vi "sequence_edited2.vi"() -> ()   [LabVIEW 2020]
uses:
  C:/Users/Public/Documents/Photometrics/PMQI-LabViewSamples/Examples/2018/Dependencies/PVCamNET.dll
  Dependencies/PVCamNET.dll
panel:
  in  "Trigger In Behaviour":string(combo)
  in  "Trigger Out Behaviour":string(combo)
  in  "Path":path
  out "SavingPath":string
  out "Boolean":bool
  in  "?":bool
  out "Capturing":bool
  in  "?":bool
  in  "FramesToCapture":u16
  in  "Exposure":u32
  in  "?":bool
  # "Description:\nThis code lets the user use sequence mode and save a TIFF image with \nthe user's preferred buffer size (framesToCapture) and exposure time. \n\nSteps to run:\n1. Update Path (Example: d:\\Temp\\ )\n2. Click \"Run\"\n3. Enter FramesToCapture and Exposure time\n4. Click \"START\"\n5. Click \"SAVE\"\n6. Click \"CLOSE\""
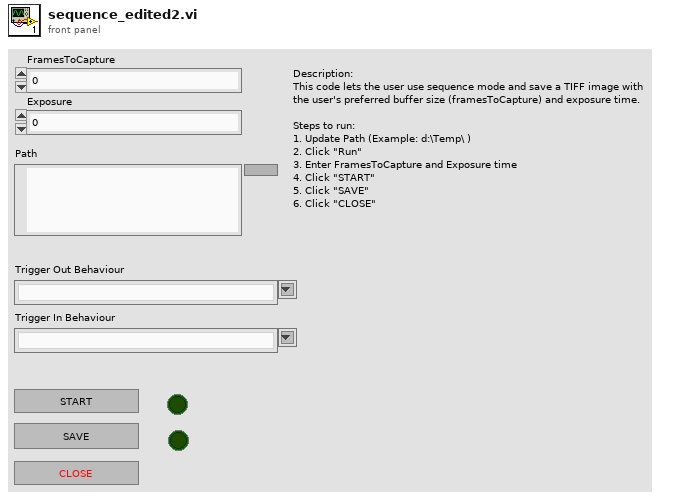
[diagram p1: front panel]
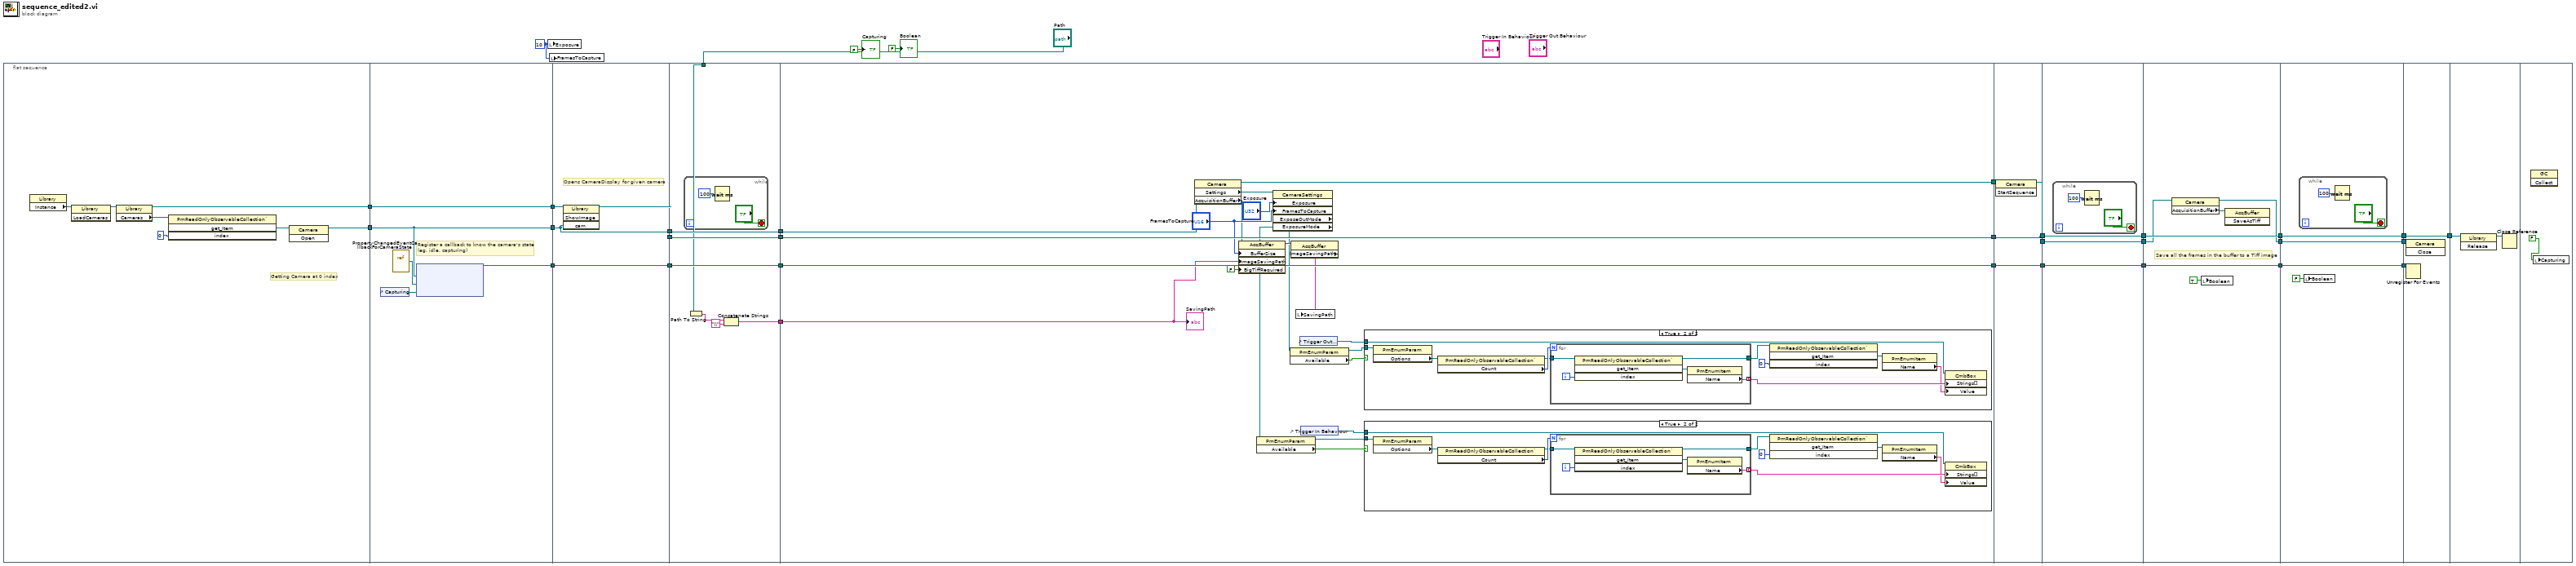
[diagram p0: block diagram]
diagram:
  w13 = u32 10 ("Exposure")
  n1 = flat-sequence {
    tunnel: [w35] -> w32
    tunnel: [w36] -> w31
    tunnel: w32 -> [w44]
    tunnel: [w44] -> w30
    tunnel: w31 -> [w41]
    tunnel: [w41] -> w29
    tunnel: [w40] -> w28
    tunnel: w30 -> [w48]
    tunnel: w29 -> [w47]
    tunnel: [w47] -> w26
    tunnel: [w46] -> w27
    tunnel: [w45] -> w25
    tunnel: w28 -> [w45]
    tunnel: w27 -> [w55]
    tunnel: [w55] -> w24
    tunnel: w26 -> [w54]
    tunnel: [w54] -> w23
    tunnel: [w53] -> w22
    tunnel: w25 -> [w53]
    tunnel: [w50] -> w2
    tunnel: "Path" -> [w49]
    tunnel: [w77] -> w21
    tunnel: [w76] -> w20
    tunnel: w24 -> [w76]
    tunnel: w23 -> [w75]
    tunnel: [w72] -> w19
    tunnel: w22 -> [w72]
    tunnel: w2 -> [w66]
    tunnel: w21 -> [w109]
    tunnel: [w108] -> w18
    tunnel: w20 -> [w111]
    tunnel: [w111] -> w17
    tunnel: [w110] -> w16
    tunnel: w19 -> [w110]
    tunnel: w18 -> [w114]
    tunnel: [w114] -> w12
    tunnel: w17 -> [w113]
    tunnel: [w113] -> w11
    tunnel: w16 -> [w112]
    tunnel: [w112] -> w10
    tunnel: w12 -> [w119]
    tunnel: [w118] -> w9
    tunnel: w11 -> [w122]
    tunnel: [w122] -> w7
    tunnel: w10 -> [w121]
    tunnel: [w121] -> w5
    tunnel: w9 -> [w126]
    tunnel: [w126] -> w8
    tunnel: w7 -> [w125]
    tunnel: [w125] -> w6
    tunnel: w5 -> [w124]
    tunnel: [w124] -> w4
    tunnel: w8 -> [w131]
    tunnel: w6 -> [w130]
    tunnel: [w130] -> w15
    tunnel: w4 -> [w129]
    tunnel: w15 -> [w133]
    frame #0 {
      # "Getting Camera at 0 index"
      n2 = property class="Library"() -> ("Instance"=w34:refnum<k24>)  [unwired: 2 in, 2 out]
      n3 = invoke class="Library" method="LoadCameras"(reference=w34) -> (reference out=w33:refnum<k24>)  [unwired: 2 in, 2 out]
      n4 = property class="Library"(reference=w33) -> (reference out=w35:refnum<k24>, "Cameras"=w39:refnum<k24>)  [unwired: 1 in, 1 out]
      n5 = invoke class="PmReadOnlyObservableCollection`" method="get_Item"(reference=w39, "index"=0) -> ("get_Item"=w37:refnum<k24>)  [unwired: 2 in, 3 out]
      n6 = invoke class="Camera" method="Open"(reference=w37) -> (reference out=w36:refnum<k24>)  [unwired: 2 in, 2 out]
    }
    frame #1 {
      # "Register a callback to know the camera's state \n(eg. idle, capturing)"
      n7 = control-ref of="Capturing"() -> (w43:refnum<vi>)
      n8 = vi-ref "PropertyChangedEventCallbackForCameraState.vi"() -> ("vi reference"=w42:refnum<vi>)
      n9 = node(w41, w42, w43) -> (w40:refnum<k27>)  [unwired: 2 in, 1 out]
    }
    frame #2 {
      # "Opens CameraDisplay for given camera"
      n10 = invoke class="Library" method="ShowImage"(reference=w48, "cam"=w47) -> (reference out=w46:refnum<k24>)  [unwired: 2 in, 3 out]
    }
    frame #3 {
      n11 = while {
        stop <- "?" stop-if-true
        n12 = Wait (ms)(milliseconds to wait=u32 100) -> ()  [unwired: 1 out]
      }
      n13 = Path To String(path=w49) -> (string=w52:string)
      n14 = Concatenate Strings(w52, "\\" ("string")) -> (w50:string)
    }
    frame #4 {
      n15 = property class="Camera"(reference=w75) -> (reference out=w77:refnum<k24>, "Settings"=w74:refnum<k24>, "AcquisitionBuffer"=w70:refnum<k24>)  [unwired: 1 in, 1 out]
      n16 = property class="AcqBuffer"(reference=w70, "BufferSize"="FramesToCapture", "ImageSavingPath"=w66, "BigTiffRequired"=FALSE) -> (reference out=w69:refnum<k24>)  [unwired: 1 in, 1 out]
      n17 = property class="CameraSettings"(reference=w74, "Exposure"="Exposure", "FramesToCapture"="FramesToCapture") -> ("ExposeOutMode"=w59:refnum<k24>, "ExposureMode"=w58:refnum<k24>)  [unwired: 1 in, 2 out]
      n18 = property class="PmEnumParam"(reference=w58) -> (reference out=w62:refnum<k24>, "Available"=w61:bool)  [unwired: 1 in, 1 out]
      n19 = property class="PmEnumParam"(reference=w59) -> (reference out=w65:refnum<k24>, "Available"=w64:bool)  [unwired: 1 in, 1 out]
      n20 = property class="AcqBuffer"(reference=w69) -> ("ImageSavingPath"=w67:string)  [unwired: 1 in, 2 out]
      n21 = local write "SavingPath"(w67) -> ()
      n22 = control-ref of="Trigger Out Behaviour"() -> (w63:refnum<vi>)
      n23 = control-ref of="Trigger In Behaviour"() -> (w60:refnum<vi>)
      n24 = case shown="True" w64 {
        tunnel: w65 -> [_ w102]
        tunnel: w63 -> [_ w93]
        frame False {
        }
        frame True {
          n25 = property class="PmEnumParam"(reference=w102) -> ("Options"=w101:refnum<k24>)  [unwired: 1 in, 2 out]
          n26 = property class="PmReadOnlyObservableCollection`"(reference=w101) -> (reference out=w99:refnum<k24>, "Count"=w100:i32)  [unwired: 1 in, 1 out]
          n27 = for {
            N: w100 -> [_]
            tunnel: w99 -> [w107]
            tunnel: [w104] -> w96
            tunnel: [w103] -> w95 mode=indexing
            i -> [w106]
            n28 = invoke class="PmReadOnlyObservableCollection`" method="get_Item"(reference=w107, "index"=w106) -> (reference out=w104:refnum<k24>, "get_Item"=w105:refnum<k24>)  [unwired: 2 in, 2 out]
            n29 = property class="PmEnumItem"(reference=w105) -> ("Name"=w103:string)  [unwired: 1 in, 2 out]
          }
          n30 = invoke class="PmReadOnlyObservableCollection`" method="get_Item"(reference=w96, "index"=0) -> ("get_Item"=w97:refnum<k24>)  [unwired: 2 in, 3 out]
          n31 = property class="PmEnumItem"(reference=w97) -> ("Name"=w94:string)  [unwired: 1 in, 2 out]
          n32 = property class="CmbBox"(reference=w93, "Strings[]"=w95, "Value"=w94) -> ()  [unwired: 1 in, 2 out]
        }
      }
      n33 = case shown="True" w61 {
        tunnel: w62 -> [_ w87]
        tunnel: w60 -> [_ w78]
        frame False {
        }
        frame True {
          n34 = property class="PmEnumParam"(reference=w87) -> ("Options"=w86:refnum<k24>)  [unwired: 1 in, 2 out]
          n35 = property class="PmReadOnlyObservableCollection`"(reference=w86) -> (reference out=w84:refnum<k24>, "Count"=w85:i32)  [unwired: 1 in, 1 out]
          n36 = for {
            N: w85 -> [_]
            tunnel: w84 -> [w92]
            tunnel: [w89] -> w83
            tunnel: [w88] -> w80 mode=indexing
            i -> [w91]
            n37 = invoke class="PmReadOnlyObservableCollection`" method="get_Item"(reference=w92, "index"=w91) -> (reference out=w89:refnum<k24>, "get_Item"=w90:refnum<k24>)  [unwired: 2 in, 2 out]
            n38 = property class="PmEnumItem"(reference=w90) -> ("Name"=w88:string)  [unwired: 1 in, 2 out]
          }
          n39 = invoke class="PmReadOnlyObservableCollection`" method="get_Item"(reference=w83, "index"=0) -> ("get_Item"=w81:refnum<k24>)  [unwired: 2 in, 3 out]
          n40 = property class="PmEnumItem"(reference=w81) -> ("Name"=w79:string)  [unwired: 1 in, 2 out]
          n41 = property class="CmbBox"(reference=w78, "Strings[]"=w80, "Value"=w79) -> ()  [unwired: 1 in, 2 out]
        }
      }
      "SavingPath" <- w66
    }
    frame #5 {
      n42 = invoke class="Camera" method="StartSequence"(reference=w109) -> (reference out=w108:refnum<k24>)  [unwired: 2 in, 2 out]
    }
    frame #6 {
      n43 = while {
        stop <- "?" stop-if-true
        n44 = Wait (ms)(milliseconds to wait=u32 100) -> ()  [unwired: 1 out]
      }
    }
    frame #7 {
      # "Save all the frames in the buffer to a Tiff image"
      n45 = property class="Camera"(reference=w119) -> (reference out=w118:refnum<k24>, "AcquisitionBuffer"=w120:refnum<k24>)  [unwired: 1 in, 1 out]
      n46 = local write "Boolean"(TRUE ("Boolean")) -> ()
      n47 = invoke class="AcqBuffer" method="SaveAsTiff"(reference=w120) -> ()  [unwired: 2 in, 3 out]
    }
    frame #8 {
      n48 = while {
        stop <- "?" stop-if-true
        n49 = Wait (ms)(milliseconds to wait=u32 100) -> ()  [unwired: 1 out]
      }
      n50 = local write "Boolean"(FALSE ("Boolean")) -> ()
    }
    frame #9 {
      n51 = invoke class="Camera" method="Close"(reference=w131) -> ()  [unwired: 2 in, 3 out]
      n52 = Unregister For Events(event registration refnum=w129) -> ()  [unwired: 1 in, 1 out]
    }
    frame #10 {
      n53 = invoke class="Library" method="Release"(reference=w133) -> (reference out=w132:refnum<k24>)  [unwired: 2 in, 2 out]
      n54 = Close Reference(reference=w132) -> ()  [unwired: 1 in, 1 out]
    }
    frame #11 {
      n55 = invoke class="GC" method="Collect"() -> ()  [unwired: 3 in, 3 out]
      n56 = local write "Capturing"(FALSE ("Boolean")) -> ()
    }
  }
  n57 = local write "Exposure"(w13) -> ()
  n58 = local write "FramesToCapture"(w13) -> ()
  "Capturing" <- FALSE ("Capturing")
  "Boolean" <- FALSE ("Boolean")
